vi "monochromator.vi"() -> ()   [LabVIEW 2014]
panel:
  out "Raman Wavelength":dbl
  in  "Raman Shift":dbl
  in  "Laser Wavelength":dbl
  in  "OK Button":bool
  in  "Grating number":u32
  out "Current Grating":i16=1 min=1 max=9
  in  "Change grating":bool
  in  "stop":bool
  out "Wavelength":dbl format="%.1f"
  in  "Center wavelength":dbl
  in  "Set wavelength":bool
  out "Label":string
  out "Grooves":dbl format="%.1f"
  out "error out":errorcluster
  in  "error in (no error)":errorcluster
  # "Grating information:\n1: 600 gr/mm, 750 nm blaze\n2: 300 gr/mm, 1000 nm blaze\n3.  150 gr/mm, 500 nm blaze"
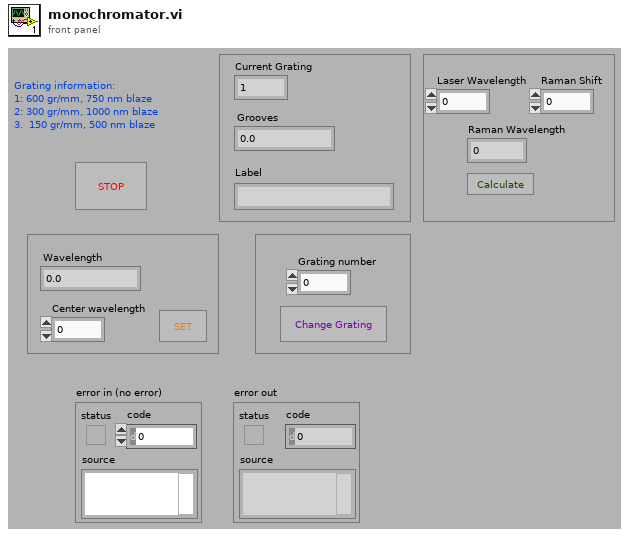
[diagram p1: front panel]
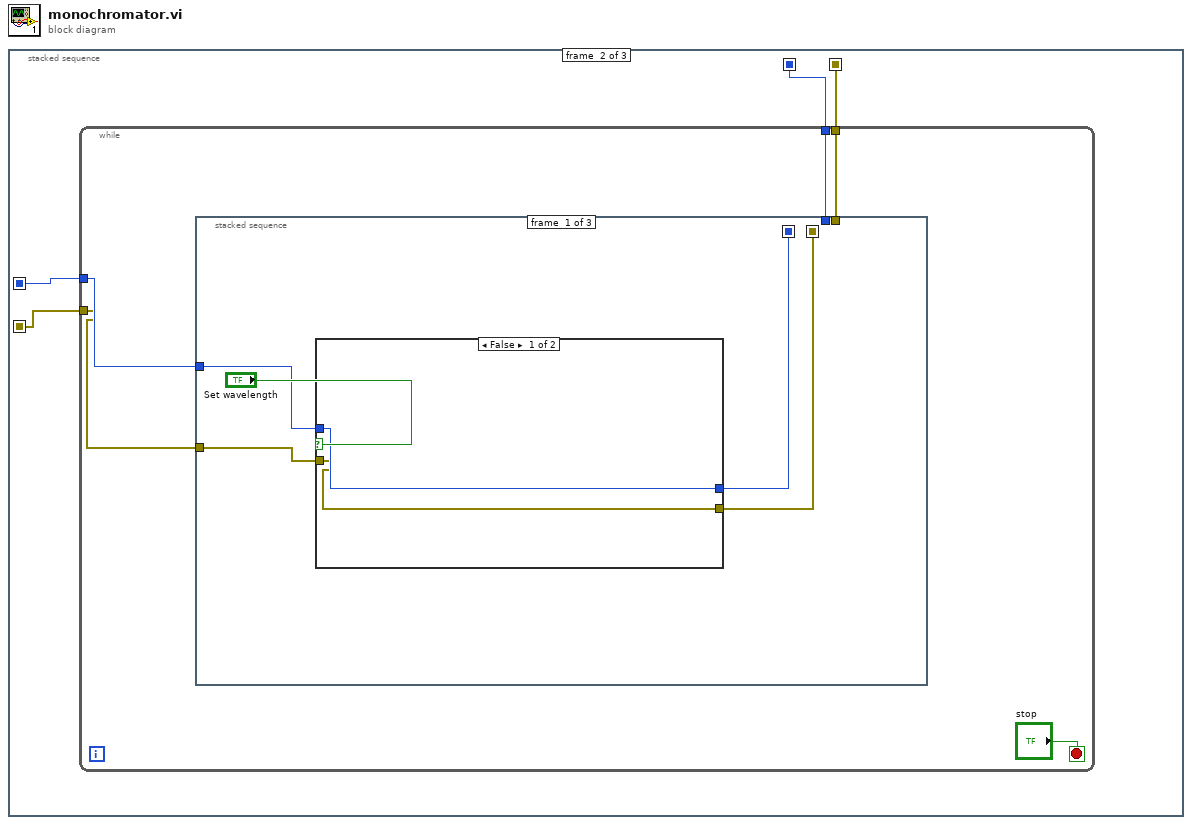
[diagram p0: block diagram]
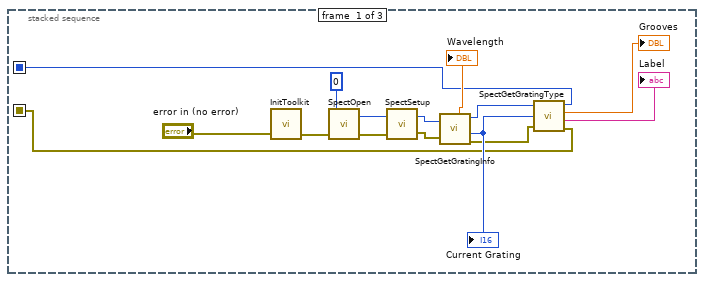
[diagram p2: hidden frame]
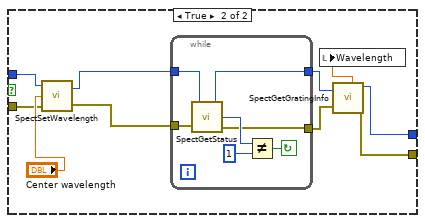
[diagram p3: hidden frame]
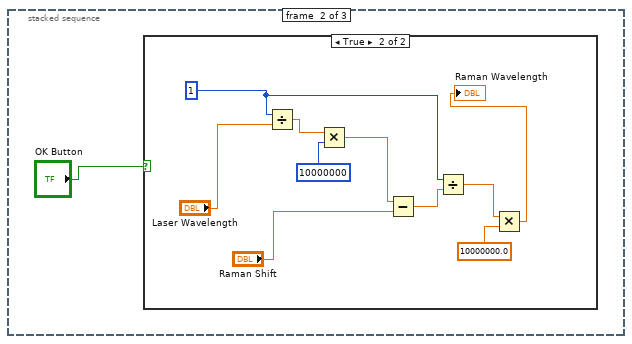
[diagram p4: hidden frame]
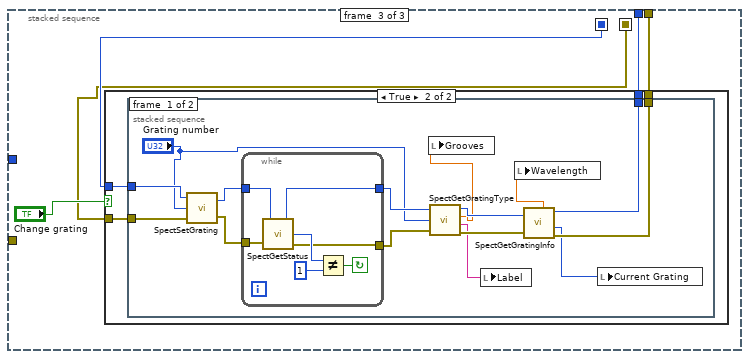
[diagram p6: hidden frame]
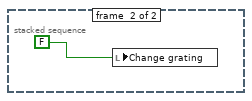
[diagram p8: hidden frame]
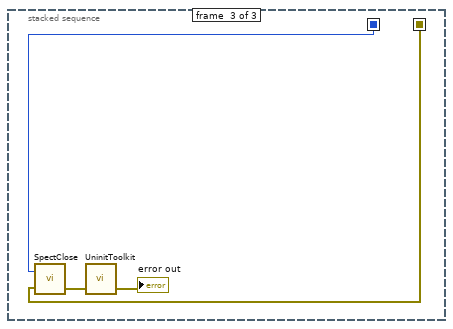
[diagram p9: hidden frame]
diagram:
  n1 = stacked-sequence {
    seq-local: [w3 _ _] -> [_ w19 _]
    seq-local: [w4 _ _] -> [_ w18 _]
    seq-local: [_ w17 _] -> [_ _ w95]
    seq-local: [_ w16 _] -> [_ _ w94]
    frame #0 {
      n2 = call <userlib>:"InitToolkit.vi"("error in"="error in (no error)") -> ("error out"=w14:errorcluster)
      n3 = call <userlib>:"SpectOpen.vi"("error in"=w14, "Spectrometer ID"=0) -> ("error out"=w13:errorcluster, "Spectrometer Handle"=w11:u32)  [unwired: 1 in]
      n4 = call <userlib>:"SpectSetup.vi"("error in"=w13, "Spectrometer Handle"=w11) -> ("error out"=w2:errorcluster, "Spectrometer Handle"=w1:u32)
      n5 = call <userlib>:"SpectGetGratingInfo.vi"("Spectrometer Handle"=w1, "error in"=w2) -> ("Current Wavelength"=→"Wavelength":dbl, "Spectrometer Handle"=w8:u32, "Current Grating"=w9:i16, "error out"=w7:errorcluster)  [unwired: 2 out]
      "Current Grating" <- w9
      n6 = call <userlib>:"SpectGetGratingType.vi"("Spectrometer Handle"=w8, "Grating Number"=w9, "error in"=w7) -> ("Spectrometer Handle"=w3:u32, "Grooves per mm"=→"Grooves":dbl, "Label"=→"Label":string, "error out"=w4:errorcluster)
    }
    frame #1 {
      n7 = while {
        tunnel: w19 -> [w23]
        tunnel: w18 -> [w22]
        tunnel: [w21] -> w17
        tunnel: [w20] -> w16
        stop <- "stop" stop-if-true
        n8 = stacked-sequence {
          seq-local: [w26 _ _] -> [_ _ w63]
          seq-local: [w25 _ _] -> [_ _ w62]
          tunnel: w23 -> [w28 _ _]
          tunnel: w22 -> [w27 _ _]
          tunnel: [_ _ w61] -> w21
          tunnel: [_ _ w60] -> w20
          frame #0 {
            n9 = case shown="False" "Set wavelength" {
              tunnel: [w30 w35] -> w25
              tunnel: [w31 w34] -> w26
              tunnel: w28 -> [w31 w33]
              tunnel: w27 -> [w30 w32]
              frame False {
              }
              frame True {
                n10 = call <userlib>:"SpectSetWavelength.vi"("error in"=w32, "Wavelength"="Center wavelength", "Spectrometer Handle"=w33) -> ("error out"=w39:errorcluster, "Spectrumeter Handle"=w40:u32)
                n11 = while {
                  tunnel: w40 -> [w45]
                  tunnel: w39 -> [w44]
                  tunnel: [w43] -> w37
                  tunnel: [w42] -> w36
                  stop <- w46 continue-if-true
                  n12 = call <userlib>:"SpectGetStatus.vi"("Spectrometer Handle"=w45, "error in"=w44) -> ("Spectrometer Handle"=w43:u32, "Command Status"=w47:u32, "error out"=w42:errorcluster)
                  n13 = Not Equal?(x=w47, y=u32 1) -> (x != y?=w46:bool)
                }
                n14 = call <userlib>:"SpectGetGratingInfo.vi"("Spectrometer Handle"=w37, "error in"=w36) -> ("Current Wavelength"=w38:dbl, "Spectrometer Handle"=w34:u32, "error out"=w35:errorcluster)  [unwired: 3 out]
                n15 = local write "Wavelength"(w38) -> ()
              }
            }
          }
          frame #1 {
            n16 = case shown="True" "OK Button" {
              frame False {
              }
              frame True {
                w54 = 1
                n17 = Divide(x=w54, y="Laser Wavelength") -> (x/y=w57:dbl)
                n18 = Multiply(x=w57, y=10000000) -> (x*y=w56:dbl)
                n19 = Subtract(x=w56, y="Raman Shift") -> (x-y=w53:dbl)
                n20 = Divide(x=w54, y=w53) -> (x/y=w52:dbl)
                n21 = Multiply(x=w52, y=10000000.0) -> (x*y=→"Raman Wavelength":dbl)
              }
            }
          }
          frame #2 {
            n22 = case shown="True" "Change grating" {
              tunnel: w63 -> [w66 w70]
              tunnel: w62 -> [w65 w69]
              tunnel: [w66 w68] -> w61
              tunnel: [w65 w67] -> w60
              frame False {
              }
              frame True {
                n23 = stacked-sequence {
                  tunnel: w70 -> [w79 _]
                  tunnel: w69 -> [w78 _]
                  tunnel: [w77 _] -> w68
                  tunnel: [w76 _] -> w67
                  frame #0 {
                    n24 = call <userlib>:"SpectSetGrating.vi"("error in"=w78, "Grating Number"="Grating number", "Sepctrometer Handle"=w79) -> ("error out"=w84:errorcluster, "Spectrometer Handle"=w85:u32)
                    n25 = while {
                      tunnel: w85 -> [w89]
                      tunnel: w84 -> [w88]
                      tunnel: [w87] -> w83
                      tunnel: [w86] -> w82
                      stop <- w90 continue-if-true
                      n26 = call <userlib>:"SpectGetStatus.vi"("Spectrometer Handle"=w89, "error in"=w88) -> ("Spectrometer Handle"=w87:u32, "Command Status"=w91:u32, "error out"=w86:errorcluster)
                      n27 = Not Equal?(x=w91, y=u32 1) -> (x != y?=w90:bool)
                    }
                    n28 = call <userlib>:"SpectGetGratingType.vi"("Spectrometer Handle"=w83, "Grating Number"="Grating number", "error in"=w82) -> ("Spectrometer Handle"=w81:u32, "Grooves per mm"=w74:dbl, "Label"=w73:string, "error out"=w80:errorcluster)
                    n29 = local write "Grooves"(w74) -> ()
                    n30 = local write "Label"(w73) -> ()
                    n31 = call <userlib>:"SpectGetGratingInfo.vi"("Spectrometer Handle"=w81, "error in"=w80) -> ("Current Wavelength"=w75:dbl, "Spectrometer Handle"=w77:u32, "Current Grating"=w72:i16, "error out"=w76:errorcluster)  [unwired: 2 out]
                    n32 = local write "Wavelength"(w75) -> ()
                    n33 = local write "Current Grating"(w72) -> ()
                  }
                  frame #1 {
                    n34 = local write "Change grating"(FALSE) -> ()
                  }
                }
              }
            }
          }
        }
      }
    }
    frame #2 {
      n35 = call <userlib>:"SpectClose.vi"("error in"=w94, "Spectrometer Handle"=w95) -> ("error out"=w97:errorcluster)
      n36 = call <userlib>:"UninitToolkit.vi"("error in"=w97) -> ("error out"=→"error out":errorcluster)
    }
  }
